vi "data_points.vi"() -> ()   [LabVIEW 2020]
panel:
  in  "file path (use dialog)":path
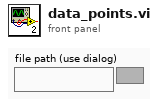
[diagram p1: front panel]
types:
  T1 = enum16{"open", "replace", "create", "open or create", "replace or create", "replace or create with confirmation"}
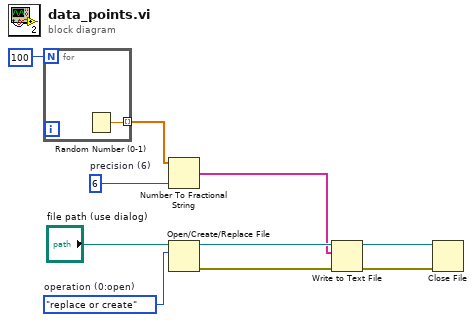
[diagram p0: block diagram]
diagram:
  w2 = i16 6  # precision (6)
  w4 = T1."replace or create"  # operation (0:open)
  n1 = for {
    N: 100 -> [_]
    tunnel: [w11] -> w3 mode=indexing
    n2 = Random Number (0-1)() -> (number: 0 to 1=w11:dbl)
  }
  n3 = Number To Fractional String(number=w3, precision (6)=w2) -> (F-format string=w1:string[])  [unwired: 2 in]
  n4 = Open/Create/Replace File(file path (use dialog)="file path (use dialog)", operation (0:open)=w4) -> (refnum out=w9:refnum<file>, error out=w7:errorcluster)  [unwired: 4 in, 1 out]
  n5 = Write to Text File(file (use dialog)=w9, text=w1, error in=w7) -> (refnum out=w8:refnum<file>, error out=w6:errorcluster)  [unwired: 1 in, 1 out]
  n6 = Close File(refnum=w8, error in=w6) -> ()  [unwired: 2 out]
